vi "Global Settings.vi"() -> ()   [LabVIEW 2015, in "Configuration Tool.lvlib"]
uses:
  Configuration Tool.lvlib
panel:
  in  "Target Project":path
  in  "VeriStand Version":enum16{"2013", "2014", "2015", "2016"}(ring)=enum."2015"
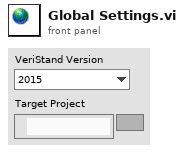
[diagram p1: front panel]
diagram:
